vi "Init Root Actors.vi"(6 "Core Actors":refnum<class "Actor.lvclass">[](array[class]), 9 "Mid Actors":refnum<class "Actor.lvclass">[](array[class]), 10 "Edge Actors":refnum<class "Actor.lvclass">[](array[class])) -> (2 "Root Actors":refnum<class "Root Actors.lvclass">)   [LabVIEW 2020, in "jettl.lvlib"]
uses:
  jettl.lvlib
  Actor/Actor.lvclass
  Root Actors/Root Actors.lvclass
  Base Root Actors/Base Root Actors.lvlib
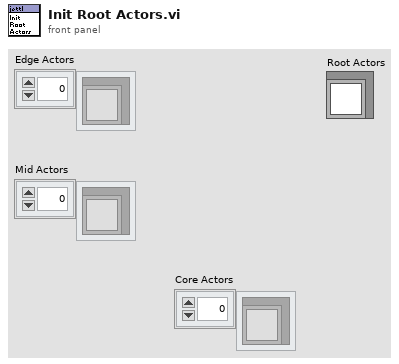
[diagram p1: front panel]
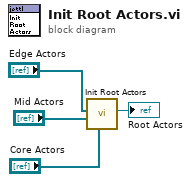
[diagram p0: block diagram]
diagram:
  n1 = call "Init Root Actors.vi"("Core Actors"="Core Actors", "Mid Actors"="Mid Actors", "Edge Actors"="Edge Actors") -> ("Root Actors"=→"Root Actors":refnum<class "Root Actors.lvclass">)  [unwired: 8 in]
